vi "MeasAction.vi"(8 "error in (no error)":errorcluster caption="entrée d'erreur (pas d'erreur)", 9 "CurvePointIndex":i32, 10 "AllPointIndex":i32, 11 "ClassData In":refnum<class "EGG5210.lvclass"> caption="DNL_LabVIEW Object in") -> (0 "error out":errorcluster caption="sortie d'erreur", 2 "MeasDatOut":dbl[](array[numeric]), 3 "ClassData Out":refnum<class "EGG5210.lvclass"> caption="DNL_LabVIEW Object out")   [LabVIEW 2012, in "EGG5210.lvclass"]
uses:
  EGG5210.lvclass
  EGG5210.lvclass/EGG5210.ctl
  <userlib>/GenProg/WritebyWeakRefBool.vi
  <vilib>/Analysis/baseanly.llb/Mean (DBL).vi
  <userlib>/GenProg/WritebyWeakRefNum.vi
  <vilib>/Analysis/NI_AALBase.lvlib
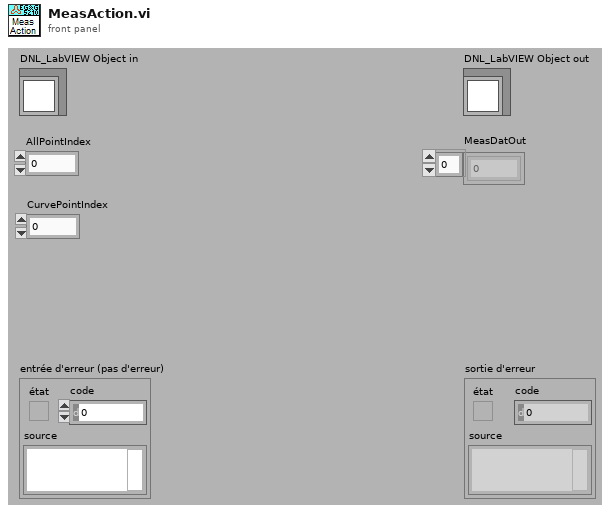
[diagram p1: front panel]
types:
  T1 = enum16{"X Output", "Y Output", "X and Y Output", "Mag", "Phase", "Mag & Phase", "X,Y,Mag & Phase", "Noise", "Aux In 1", "Aux In 2", "Aux In 3", "Aux In 4"}
  T2 = typedef "EGG5210.lvclass/EGG5210_Func.ctl" = enum16{"Read X & Y (V)", "Read Mag & Phase (V,°)", "Read X, Y, Mag & Phase (V,V,V,°)", "Read ADC Ch1 (V)", "Read ADC Ch2 (V)", "Oscillator Ctrl (Hz, mV rms)", "PL Excimer Settings (Na)"}
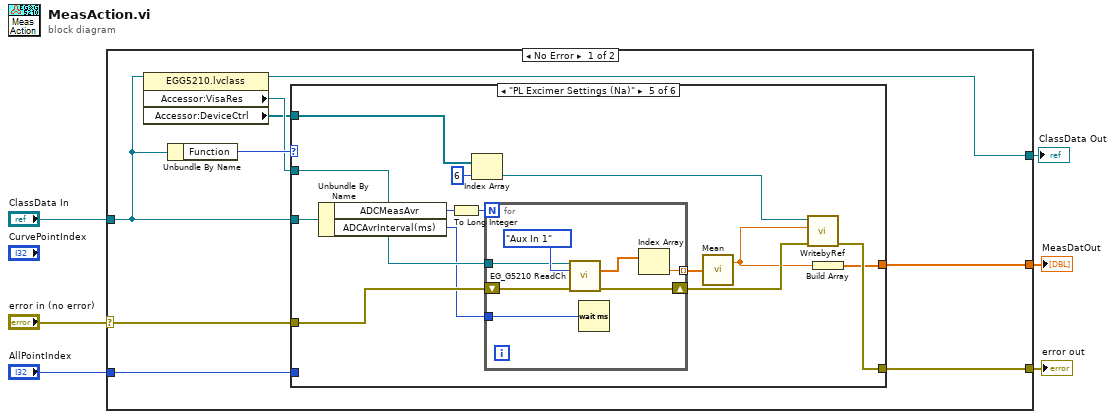
[diagram p0: block diagram]
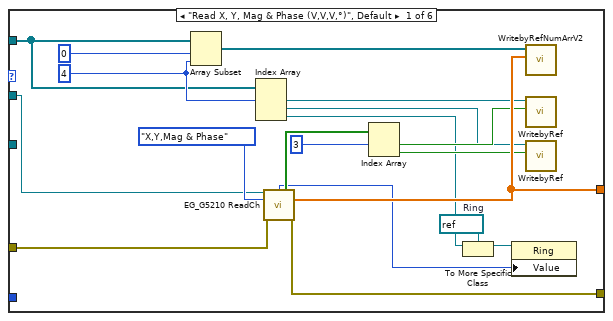
[diagram p2: hidden frame]
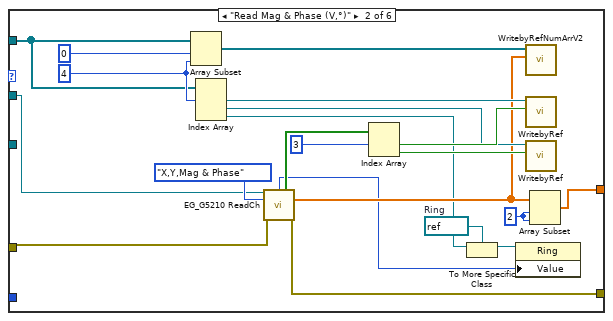
[diagram p3: hidden frame]
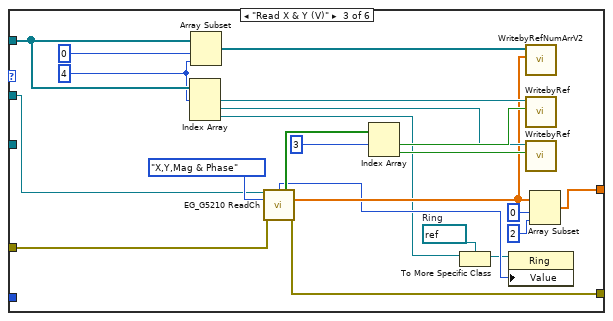
[diagram p4: hidden frame]
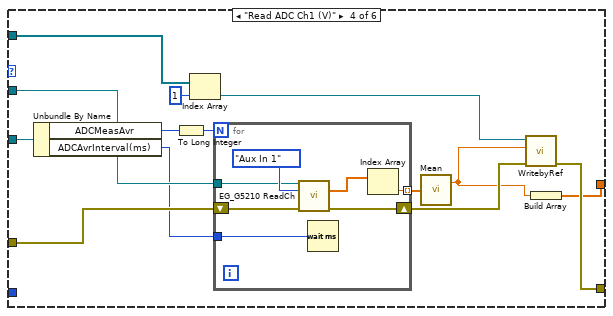
[diagram p5: hidden frame]
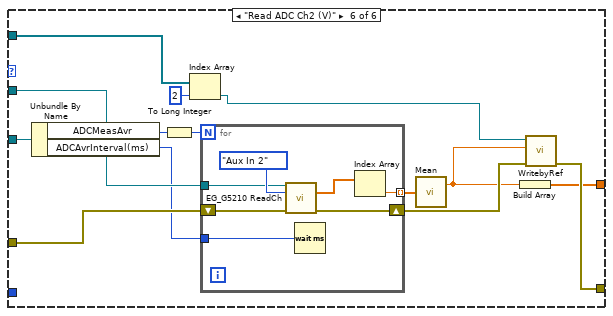
[diagram p6: hidden frame]
diagram:
  n1 = case shown="No Error" "error in (no error)" {
    selector: "error in (no error)" -> [w12 w141]
    tunnel: "ClassData In" -> [w7 w142]
    tunnel: [w10 w142] -> w4
    tunnel: "AllPointIndex" -> [w15 _]
    tunnel: [w14 w141] -> w2
    tunnel: [w13 _] -> w1
    frame No Error {
      n2 = property class="EGG5210.lvclass"(reference=w7) -> (reference out=w10:refnum<class "EGG5210.lvclass">, "Accessor:VisaRes"=w9:refnum<visa-resource-name>, "Accessor:DeviceCtrl"=w8:refnum<vi>[])  [unwired: 1 in, 1 out]
      n3 = Unbundle By Name(w7) -> ("Function"=w11:T2)
      n4 = case shown="\"PL Excimer Settings (Na)\"" w11 {
        tunnel: w15 -> [_ _ _ _ _ _]
        tunnel: [w28 w50 w72 w86 w107 w128] -> w14
        tunnel: [w30 w41 w64 w79 w100 w121] -> w13
        tunnel: w12 -> [w34 w55 w77 w85 w106 w127]
        tunnel: w9 -> [w32 w53 w75 w91 w112 w133]
        tunnel: w8 -> [w20 w42 w65 w90 w111 w132]
        tunnel: w7 -> [_ _ _ w84 w105 w126]
        frame "Read X, Y, Mag & Phase (V,V,V,°)", Default {
          w17 = refnum<vi> refnum  # Ring
          w27 = 4 ("longueur")
          n5 = Array Subset(array=w20, index=0 ("indice"), length=w27) -> (w29:refnum<vi>[])
          n6 = Index Array(array=w20, index #1=w27) -> (element #1=w24:refnum<vi>, element #2=w22:refnum<vi>, element #3=w19:refnum<vi>)  [unwired: 2 in]
          n7 = call <userlib>:"EG_G5210 ReadCh.vi"("VISA Rsrc"=w32, "Channel"=T1."X,Y,Mag & Phase", "error in (no error)"=w34) -> ("Sensitivity"=w16:u16, "Status Byte"=w26:bool[], "Outputs"=w30:dbl[], "error out"=w28:errorcluster)  [unwired: 5 in, 4 out]
          n8 = Index Array(array=w26, index #1=3 ("indice")) -> (element #1=w23:bool, element #2=w21:bool)  [unwired: 1 in]
          n9 = To More Specific Class(target class=w17, reference=w19) -> (specific class reference=w18:refnum<vi>)  [unwired: 1 in, 1 out]
          n10 = property class="Ring"(reference=w18, "Value"=w16) -> ()  [unwired: 1 in, 2 out]
          n11 = call <userlib>:"WritebyRefNumArrV2.vi"("Tableau"=w30, "Ctrl Ref"=w29) -> ()  [unwired: 9 in, 1 out]
          n12 = call-poly <userlib>:"WritebyRef.vi"("Valeur"=w23, "Control Ref"=w24) -> ()  [unwired: 9 in, 1 out]
          n13 = call-poly <userlib>:"WritebyRef.vi"("Valeur"=w21, "Control Ref"=w22) -> ()  [unwired: 9 in, 1 out]
        }
        frame "Read Mag & Phase (V,°)" {
          w36 = refnum<vi> refnum  # Ring
          w39 = 2 ("indice")
          w49 = 4 ("longueur")
          n14 = Array Subset(array=w42, index=0 ("indice"), length=w49) -> (w51:refnum<vi>[])
          n15 = Index Array(array=w42, index #1=w49) -> (element #1=w46:refnum<vi>, element #2=w44:refnum<vi>, element #3=w37:refnum<vi>)  [unwired: 2 in]
          n16 = call <userlib>:"EG_G5210 ReadCh.vi"("VISA Rsrc"=w53, "Channel"=T1."X,Y,Mag & Phase", "error in (no error)"=w55) -> ("Sensitivity"=w35:u16, "Status Byte"=w48:bool[], "Outputs"=w40:dbl[], "error out"=w50:errorcluster)  [unwired: 5 in, 4 out]
          n17 = Index Array(array=w48, index #1=3 ("indice")) -> (element #1=w45:bool, element #2=w43:bool)  [unwired: 1 in]
          n18 = To More Specific Class(target class=w36, reference=w37) -> (specific class reference=w38:refnum<vi>)  [unwired: 1 in, 1 out]
          n19 = property class="Ring"(reference=w38, "Value"=w35) -> ()  [unwired: 1 in, 2 out]
          n20 = call <userlib>:"WritebyRefNumArrV2.vi"("Tableau"=w40, "Ctrl Ref"=w51) -> ()  [unwired: 9 in, 1 out]
          n21 = call-poly <userlib>:"WritebyRef.vi"("Valeur"=w45, "Control Ref"=w46) -> ()  [unwired: 9 in, 1 out]
          n22 = call-poly <userlib>:"WritebyRef.vi"("Valeur"=w43, "Control Ref"=w44) -> ()  [unwired: 9 in, 1 out]
          n23 = Array Subset(array=w40, index=w39, length=w39) -> (w41:dbl[])
        }
        frame "Read X & Y (V)" {
          w57 = refnum<vi> refnum  # Ring
          w60 = 4 ("longueur")
          n24 = Index Array(array=w65, index #1=w60) -> (element #1=w69:refnum<vi>, element #2=w67:refnum<vi>, element #3=w56:refnum<vi>)  [unwired: 2 in]
          n25 = Array Subset(array=w65, index=0 ("indice"), length=w60) -> (w73:refnum<vi>[])
          n26 = call <userlib>:"EG_G5210 ReadCh.vi"("VISA Rsrc"=w75, "Channel"=T1."X,Y,Mag & Phase", "error in (no error)"=w77) -> ("Sensitivity"=w59:u16, "Status Byte"=w71:bool[], "Outputs"=w63:dbl[], "error out"=w72:errorcluster)  [unwired: 5 in, 4 out]
          n27 = Index Array(array=w71, index #1=3 ("indice")) -> (element #1=w68:bool, element #2=w66:bool)  [unwired: 1 in]
          n28 = To More Specific Class(target class=w57, reference=w56) -> (specific class reference=w58:refnum<vi>)  [unwired: 1 in, 1 out]
          n29 = property class="Ring"(reference=w58, "Value"=w59) -> ()  [unwired: 1 in, 2 out]
          n30 = call <userlib>:"WritebyRefNumArrV2.vi"("Tableau"=w63, "Ctrl Ref"=w73) -> ()  [unwired: 9 in, 1 out]
          n31 = call-poly <userlib>:"WritebyRef.vi"("Valeur"=w68, "Control Ref"=w69) -> ()  [unwired: 9 in, 1 out]
          n32 = call-poly <userlib>:"WritebyRef.vi"("Valeur"=w66, "Control Ref"=w67) -> ()  [unwired: 9 in, 1 out]
          n33 = Array Subset(array=w63, index=0 ("indice"), length=2 ("indice")) -> (w64:dbl[])
        }
        frame "Read ADC Ch1 (V)" {
          n34 = Unbundle By Name(w84) -> ("ADCMeasAvr"=w83:u32, "ADCAvrInterval(ms)"=w82:u32)
          n35 = To Long Integer(number=w83) -> (32bit integer=w78:i32)
          n36 = Index Array(array=w90, index=1 ("longueur")) -> (element=w88:refnum<vi>)
          n37 = for {
            N: w78 -> [_]
            tunnel: w91 -> [w97]
            tunnel: [w94] -> w81 mode=indexing
            shift-right: [w95] -> w87
            shift-left: w85 -> [w93]
            tunnel: w82 -> [w92]
            n38 = call <userlib>:"EG_G5210 ReadCh.vi"("VISA Rsrc"=w97, "Channel"=T1."Aux In 1", "error in (no error)"=w93) -> ("Outputs"=w96:dbl[], "error out"=w95:errorcluster)  [unwired: 5 in, 6 out]
            n39 = Wait (ms)(milliseconds to wait=w92) -> ()  [unwired: 1 out]
            n40 = Index Array(array=w96) -> (element=w94:dbl)  [unwired: 1 in]
          }
          n41 = call-poly <vilib>:"Mean.vi"("X"=w81) -> ("mean"=w80:dbl)  [unwired: 1 out]
          n42 = call-poly <userlib>:"WritebyRef.vi"("error in"=w87, "Valeur"=w80, "Control Ref"=w88) -> ("error out"=w86:errorcluster)  [unwired: 8 in]
          n43 = Build Array(w80) -> (w79:dbl[])
        }
        frame "PL Excimer Settings (Na)" {
          n44 = Unbundle By Name(w105) -> ("ADCMeasAvr"=w104:u32, "ADCAvrInterval(ms)"=w103:u32)
          n45 = To Long Integer(number=w104) -> (32bit integer=w99:i32)
          n46 = Index Array(array=w111, index=6 ("longueur")) -> (element=w109:refnum<vi>)
          n47 = for {
            N: w99 -> [_]
            tunnel: w112 -> [w118]
            tunnel: [w115] -> w102 mode=indexing
            shift-right: [w116] -> w108
            shift-left: w106 -> [w114]
            tunnel: w103 -> [w113]
            n48 = call <userlib>:"EG_G5210 ReadCh.vi"("VISA Rsrc"=w118, "Channel"=T1."Aux In 1", "error in (no error)"=w114) -> ("Outputs"=w117:dbl[], "error out"=w116:errorcluster)  [unwired: 5 in, 6 out]
            n49 = Wait (ms)(milliseconds to wait=w113) -> ()  [unwired: 1 out]
            n50 = Index Array(array=w117) -> (element=w115:dbl)  [unwired: 1 in]
          }
          n51 = call-poly <vilib>:"Mean.vi"("X"=w102) -> ("mean"=w101:dbl)  [unwired: 1 out]
          n52 = call-poly <userlib>:"WritebyRef.vi"("error in"=w108, "Valeur"=w101, "Control Ref"=w109) -> ("error out"=w107:errorcluster)  [unwired: 8 in]
          n53 = Build Array(w101) -> (w100:dbl[])
        }
        frame "Read ADC Ch2 (V)" {
          n54 = Unbundle By Name(w126) -> ("ADCMeasAvr"=w125:u32, "ADCAvrInterval(ms)"=w124:u32)
          n55 = To Long Integer(number=w125) -> (32bit integer=w120:i32)
          n56 = Index Array(array=w132, index=2 ("longueur")) -> (element=w130:refnum<vi>)
          n57 = for {
            N: w120 -> [_]
            tunnel: w133 -> [w139]
            tunnel: [w136] -> w123 mode=indexing
            shift-right: [w137] -> w129
            shift-left: w127 -> [w135]
            tunnel: w124 -> [w134]
            n58 = call <userlib>:"EG_G5210 ReadCh.vi"("VISA Rsrc"=w139, "Channel"=T1."Aux In 2", "error in (no error)"=w135) -> ("Outputs"=w138:dbl[], "error out"=w137:errorcluster)  [unwired: 5 in, 6 out]
            n59 = Wait (ms)(milliseconds to wait=w134) -> ()  [unwired: 1 out]
            n60 = Index Array(array=w138) -> (element=w136:dbl)  [unwired: 1 in]
          }
          n61 = call-poly <vilib>:"Mean.vi"("X"=w123) -> ("mean"=w122:dbl)  [unwired: 1 out]
          n62 = Build Array(w122) -> (w121:dbl[])
          n63 = call-poly <userlib>:"WritebyRef.vi"("error in"=w129, "Valeur"=w122, "Control Ref"=w130) -> ("error out"=w128:errorcluster)  [unwired: 8 in]
        }
      }
    }
    frame Error {
    }
  }
  "error out" <- w2
  "ClassData Out" <- w4
  "MeasDatOut" <- w1
